vi "Laser Timing Visualization.vi"() -> ()   [LabVIEW 2018]
uses:
  <vilib>/Analysis/baseanly.llb/Mean (DBL).vi
  <vilib>/Analysis/NI_AALBase.lvlib
panel:
  in  "Clear":bool
  in  "stop":bool
  out "Beam Profile":cluster{dbl[], dbl[]}(graph)={[200.0, 3000200.0, 6000200.0, 9000200.0], [454.90150356292725, 454.5925512313843, 454.8115167617798, 453.45909881591797]}
  out "Peak Vs Time":cluster{timestamp[], dbl[]}(graph)={[timestamp(3625501988.7981534 s since 1904-01-01), timestamp(3625502002.344508 s since 1904-01-01), timestamp(3625502008.385112 s since 1904-01-01), timestamp(3625502016.675941 s since 1904-01-01), timestamp(3625502023.472621 s since 1904-01-01), timestamp(3625502032.515525 s since 1904-01-01), timestamp(3625502052.062479 s since 1904-01-01)], [1100.0, 500.0, 500.0, 500.0, 200.0, 200.0, 200.0]}
  in  "Experiment name":string="Imaging"
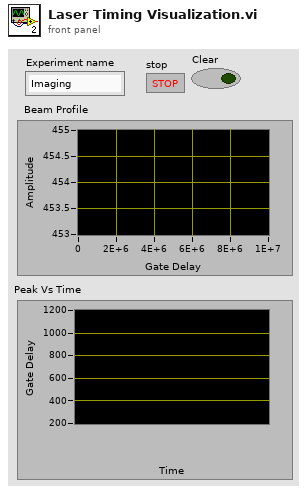
[diagram p1: front panel]
types:
  T1 = cluster{"Image":dbl[][][], "Gate Start":dbl, "Gate Width":dbl}
  T2 = cluster{"Image":dbl[][][], "Gate Start":dbl, "Gate Width":dbl}[]
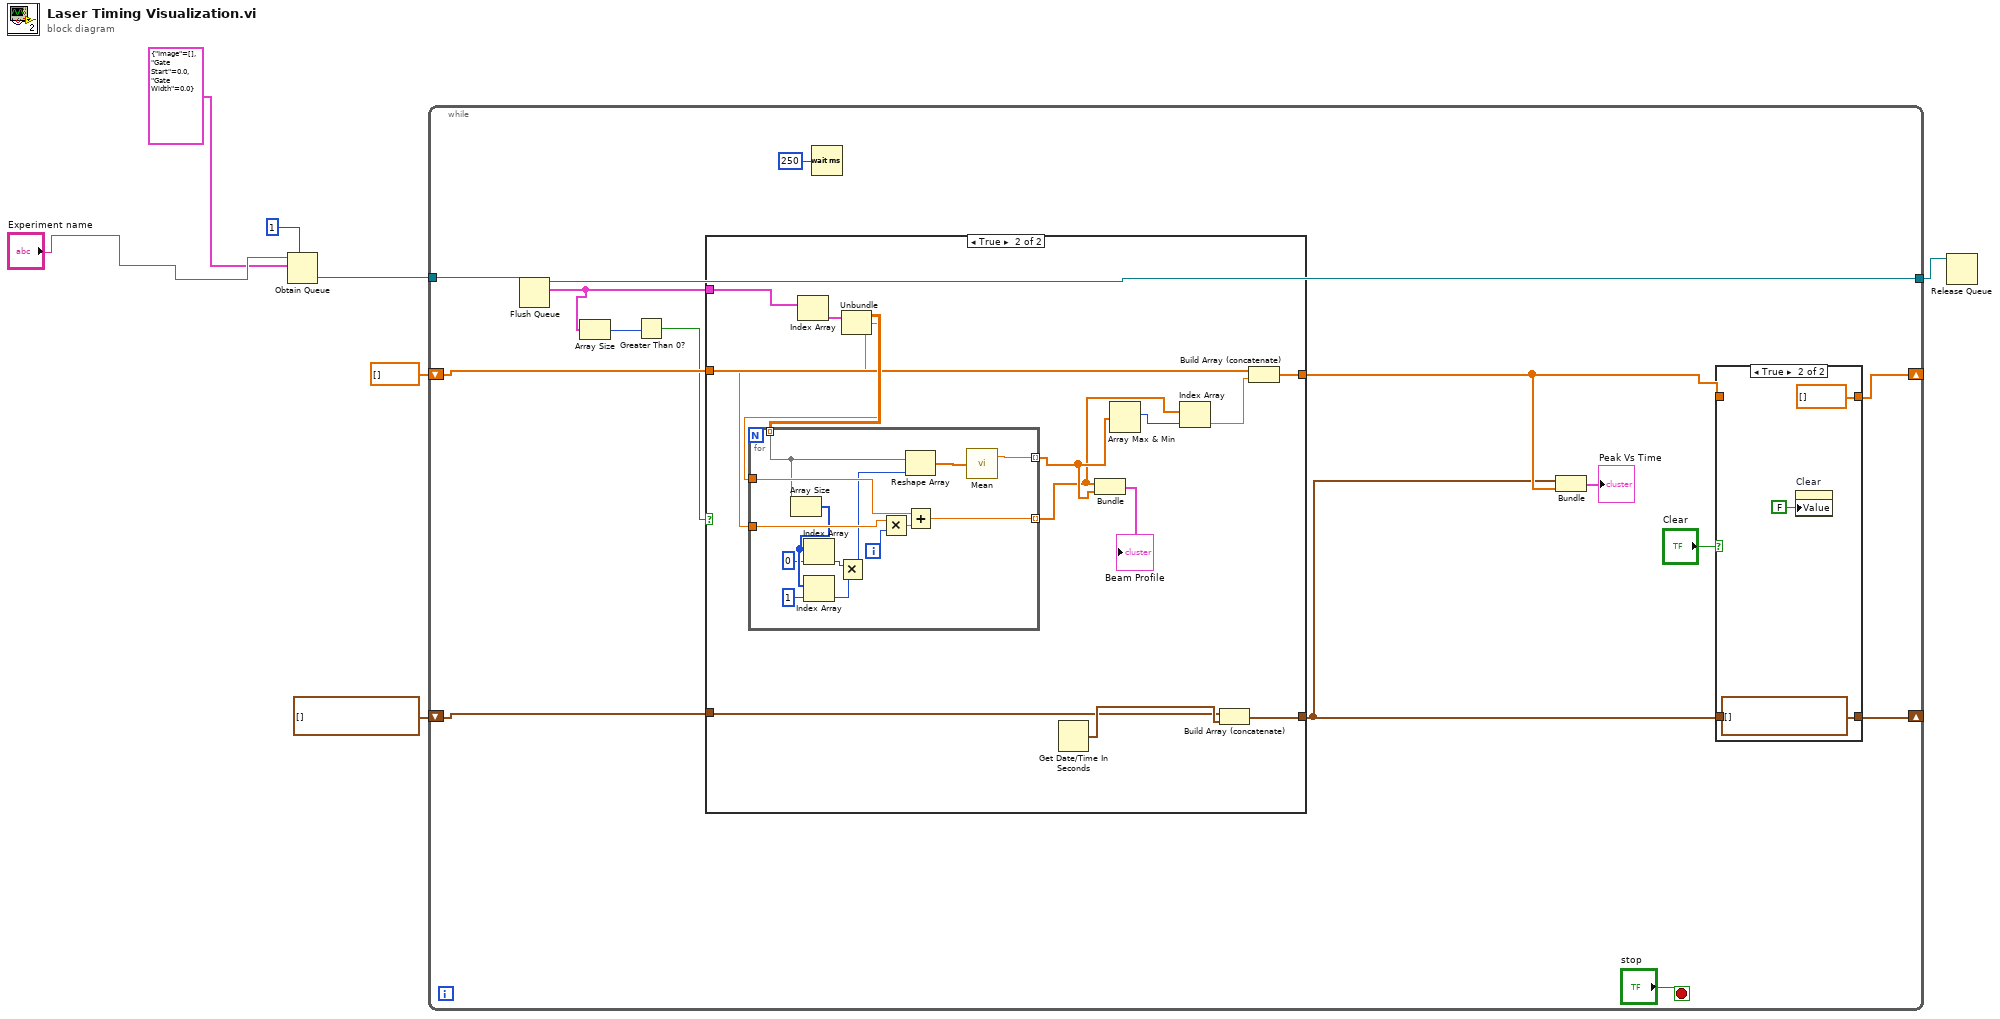
[diagram p0: block diagram]
diagram:
  n1 = Obtain Queue(max queue size (-1, unlimited)=1, name (unnamed)="Experiment name", element data type=T1 {"Image"=[], "Gate Start"=0.0, "Gate Width"=0.0} ("output cluster")) -> (queue out=w7:refnum<queue>)  [unwired: 2 in, 2 out]
  n2 = while {
    tunnel: w7 -> [w22]
    tunnel: [w21] -> w6
    shift-right: [w13] -> _
    shift-left: dbl[] [] -> [w19]
    shift-right: [w12] -> _
    shift-left: timestamp[] [] -> [w18]
    stop <- "stop" stop-if-true
    n3 = Flush Queue(queue=w22) -> (queue out=w21:refnum<queue>, remaining elements=w16:T2)  [unwired: 1 in, 1 out]
    n4 = Array Size(array=w16) -> (size(s)=w15:i32)
    n5 = Greater Than 0?(x=w15) -> (x > 0?=w14:bool)
    n6 = case shown="True" w14 {
      tunnel: w19 -> [w29 w40]
      tunnel: w18 -> [w28 w38]
      tunnel: [w29 w37] -> w9
      tunnel: [w28 w36] -> w8
      tunnel: w16 -> [_ w32]
      frame False {
      }
      frame True {
        n7 = Index Array(array=w32) -> (element=w44:T1)  [unwired: 1 in]
        n8 = Unbundle(w44) -> ("Image"=w43:dbl[][][], "Gate Start"=w34:dbl, "Gate Width"=w33:dbl)
        n9 = for {
          tunnel: w43 -> [w51] mode=indexing
          tunnel: [w58] -> w31 mode=indexing
          tunnel: w34 -> [w54]
          tunnel: w33 -> [w56]
          tunnel: [w53] -> w30 mode=indexing
          i -> [w57]
          n10 = Array Size(array=w51) -> (size(s)=w50:i32[])
          n11 = Index Array(array=w50, index=0) -> (element=w47:i32)
          n12 = Index Array(array=w50, index=1) -> (element=w46:i32)
          n13 = Multiply(x=w47, y=w46) -> (x*y=w45:i32)
          n14 = Multiply(x=w56, y=w57) -> (x*y=w55:dbl)
          n15 = Reshape Array(w51, w45) -> (w52:dbl[])
          n16 = Add(x=w54, y=w55) -> (x+y=w53:dbl)
          n17 = call-poly <vilib>:"Mean.vi"("X"=w52) -> ("mean"=w58:dbl)  [unwired: 1 out]
        }
        n18 = Get Date/Time In Seconds() -> (seconds since 1Jan1904=w39:timestamp)
        n19 = Bundle(w30, w31) -> (→"Beam Profile":cluster{dbl[], dbl[]})  [unwired: 1 in]
        n20 = Array Max & Min(array=w31) -> (max index (indices)=w42:i32)  [unwired: 3 out]
        n21 = Index Array(array=w30, index=w42) -> (element=w41:dbl)
        n22 = Build Array (concatenate)(w38, w39) -> (w36:timestamp[])
        n23 = Build Array (concatenate)(w40, w41) -> (w37:dbl[])
      }
    }
    n24 = Wait (ms)(milliseconds to wait=u32 250) -> ()  [unwired: 1 out]
    n25 = Bundle(w8, w9) -> (→"Peak Vs Time":cluster{timestamp[], dbl[]})  [unwired: 1 in]
    n26 = case shown="True" "Clear" {
      tunnel: w9 -> [w24 _]
      tunnel: [w24 dbl[] []] -> w13
      tunnel: w8 -> [w23 _]
      tunnel: [w23 timestamp[] []] -> w12
      frame False {
      }
      frame True {
        n27 = property on="Clear" class="Bool (strict)"("Value"=FALSE ("Clear")) -> ()  [unwired: 2 in, 2 out]
      }
    }
  }
  n28 = Release Queue(queue=w6) -> ()  [unwired: 2 in, 3 out]
